vi "Set Instrument Status Enable.vi"(8 "error in (no error)":errorcluster, 10 "INSE (0)":i32, 11 "VISA resource name":refnum<visa-resource-name>) -> (0 "error out":errorcluster, 3 "VISA resource name out":refnum<visa-resource-name>, 4 "Device Errors":cluster{"code":i32, "Text":string}[](array[cluster]))   [LabVIEW 2014, in "Stanford Research DG645 - Driver.lvlib"]
doc: "Status and Display Command: INSE i\nInstrument Error Check\n\nSet the Instrument Status Enable register to i. Bits set in this register cause INSB (in STB) to be set when the corresponding bit is set in the INSR register."
uses:
  Stanford Research DG645 - Driver.lvlib
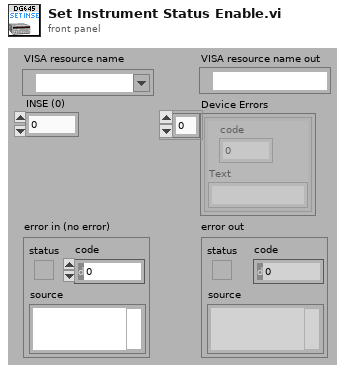
[diagram p1: front panel]
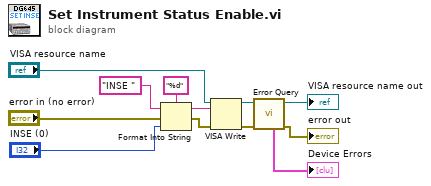
[diagram p0: block diagram]
diagram:
  n1 = Format Into String(format string="%d", initial string="INSE " ("command"), error in="error in (no error)", "INSE (0)") -> (resulting string=w9:string, error out=w10:errorcluster)
  n2 = VISA Write(VISA resource name="VISA resource name", write buffer=w9, error in (no error)=w10) -> (VISA resource name out=w4:refnum<visa-resource-name>, error out=w6:errorcluster)  [unwired: 1 out]
  n3 = call "Error Query.vi"("error in (no error)"=w6, "VISA resource name"=w4) -> ("error out"=→"error out":errorcluster, "VISA resource name out"=→"VISA resource name out":refnum<visa-resource-name>, "Device Errors"=→"Device Errors":cluster{"code":i32, "Text":string}[])  [unwired: 7 in]
